vi "GraphZoom.vi"(7 "Plot":T1 items=["FRF", "rad phase unwrapped", "deg phase unwrapped", "rad phase wrapped", "deg phase wrapped", "White Plots", "MJ Map", "Real and Imaginary"], 9 "Names":string[](array[string]), 10 "dB Range":dbl=40.0, 11 "Graph":refnum<vi>) -> ()   [LabVIEW 2022 SP3]
uses:
  <vilib>/Utility/miscctls.llb/LVPoint32TypeDef.ctl
  GraphType.ctl
panel:
  out "option":bool
  in  "rescale Y":bool
  in  "View Type":u16(ring) items=["As measured"=0, "Normalize"=1, "Cplx Average"=3, "Real Average"=4]
  in  "Send Email":bool
  in  "Rescale":bool
  in  "Copy to Clipboard":bool
  out "Position":string
  in  "offset":bool
  in  "Plot grid":u32(colorbox)=16448250
  in  "Integrate":bool
  in  "Plot background":u32(colorbox)=16448250
  in  "Matlab":bool
  in  "Plot Format":T2
  in  "Separation":dbl=1.0
  in  "Separate":bool
  in  "Slide":dbl(slide) scale=-30.0..30.0
  in  "Run":u16(ring) items=["OB23BP_Starkie 04A H.AvC", "OB23_CurtinVLA Test 03 H.AvC"]
  out "lines":i32
  out "Data":cluster{dbl, "dt":dbl, "Y":dbl[]}[](graph)
  out "XScale.NameLbl.Text":string
  out "Coords":T3
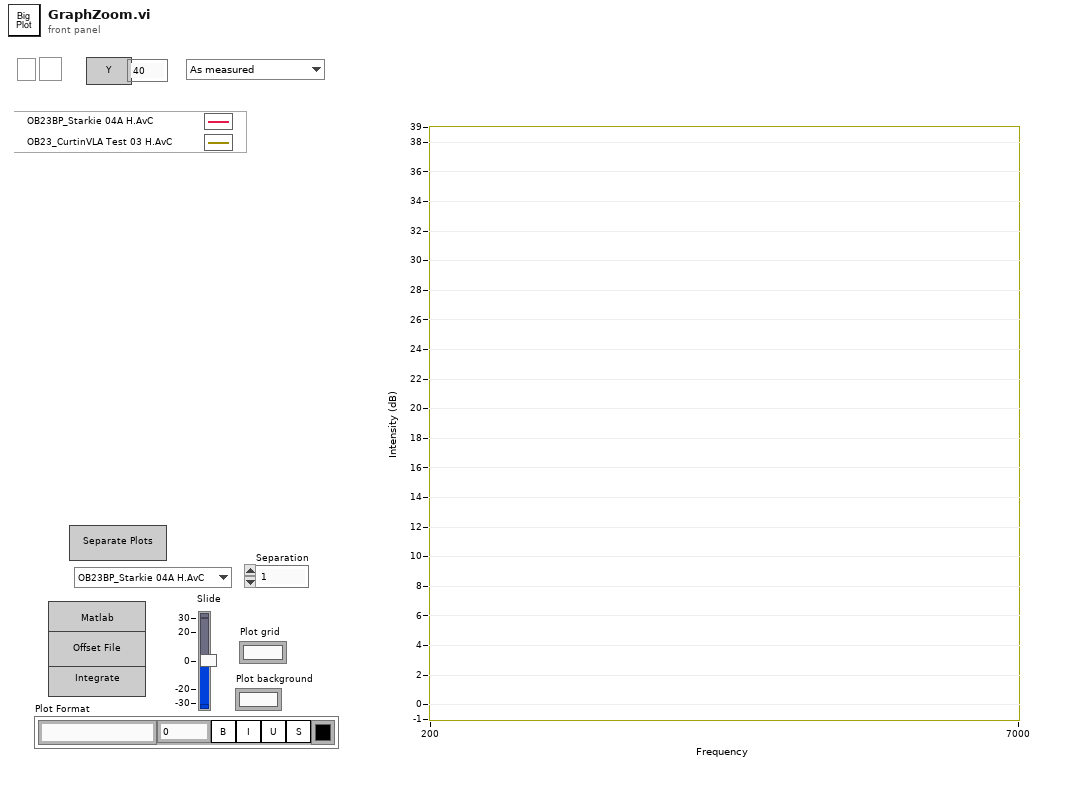
[diagram p1: front panel]
types:
  T1 = typedef "GraphType.ctl" = u16
  T2 = cluster{"Font Name":string, "Size":u16, "Bold":bool, "Italic":bool, "Underline":bool, "Strikeout":bool, "Color":u32}
  T3 = typedef "LVPoint32TypeDef.ctl" = cluster{"Horizontal":i32, "Vertical":i32}
  T4 = enum16{"Grab Lines", "Grab Bands", "Grab Centroids"}
  T5 = typedef "LVRangeTypeDef.ctl" = cluster{"Minimum":dbl, "Maximum":dbl, "Increment":dbl, "Minor Increment":dbl, "Start":dbl}
  T6 = typedef "LVFontTypeDef.ctl" = cluster{"Font Name":string, "Size":u16, "Bold":bool, "Italic":bool, "Underline":bool, "Strikeout":bool, "Color":u32}
  T7 = cluster{"View Type":u16, "Smoothing":u16, "Bands":u16, "New Band":bool, "rescale Y":bool, "rescale X":bool, "X_Low":dbl, "X_High":dbl, "dB Range":dbl, "New Band 2":bool, "X Scaling":bool, "Y Scaling":bool, "mag/phase":T1}
  T8 = cluster{"View Type":u16, "Smoothing":u16, "Bands":u16, "New Band":bool, "rescale Y":bool, "rescale X":bool, "X_Low":dbl, "X_High":dbl, "dB Range":dbl, "New Band 2":bool}
  T9 = cluster{"Shift":bool, "Ctrl":bool, "Alt":bool, "Cmd":bool, "Opt":bool}
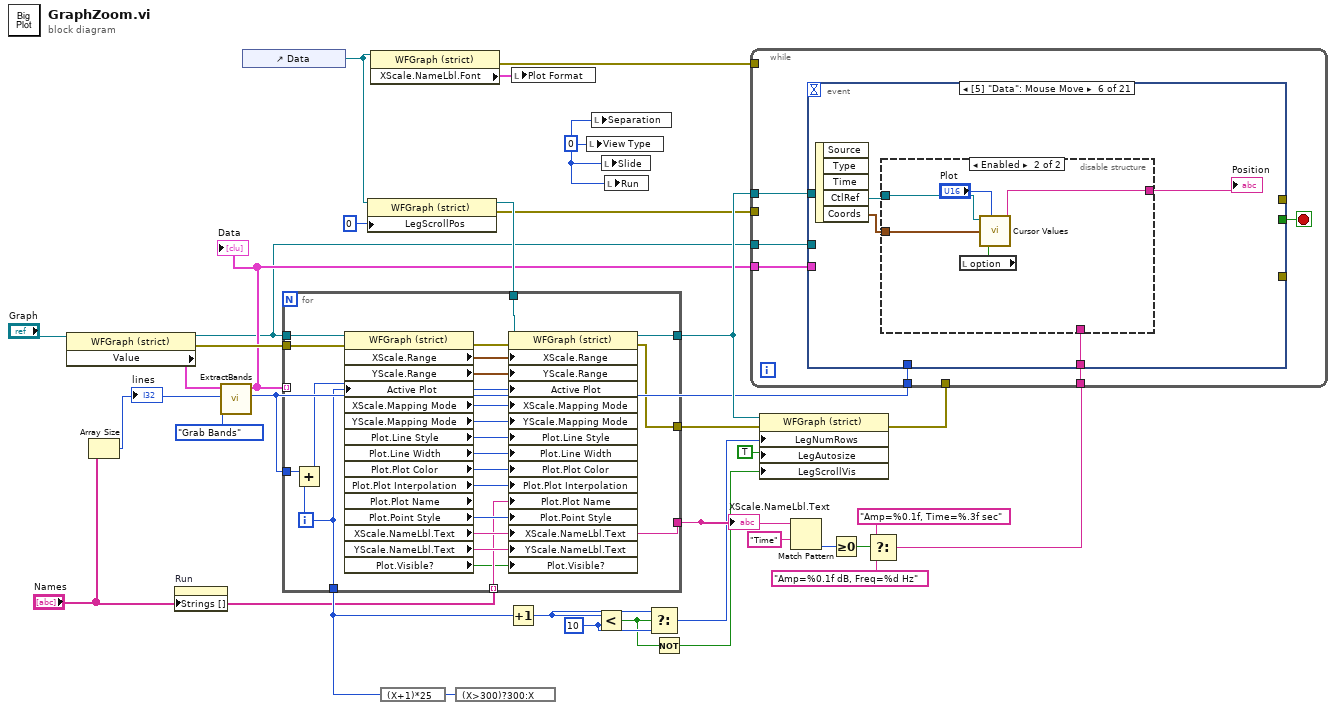
[diagram p0: block diagram]
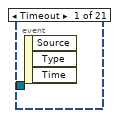
[diagram p2: hidden frame]
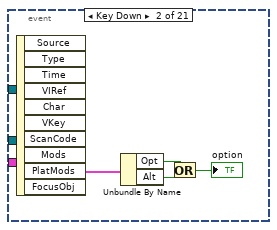
[diagram p3: hidden frame]
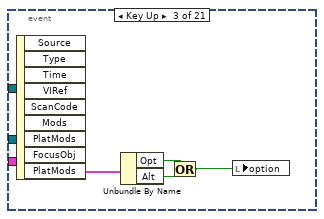
[diagram p4: hidden frame]
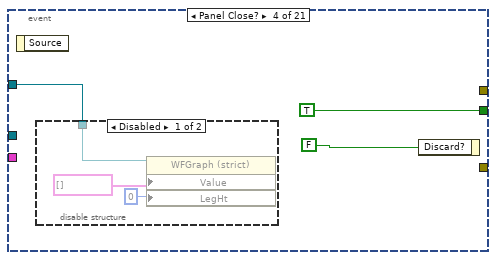
[diagram p5: hidden frame]
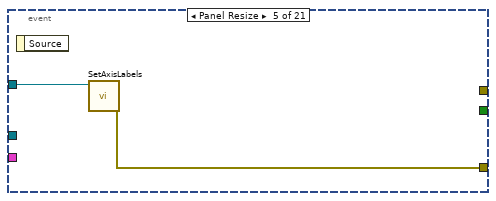
[diagram p7: hidden frame]
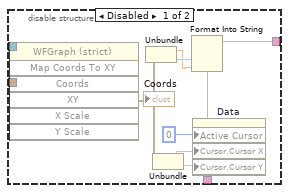
[diagram p8: hidden frame]
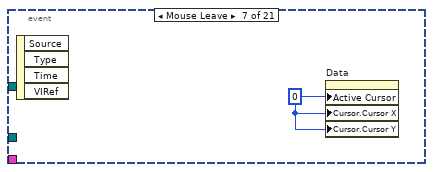
[diagram p9: hidden frame]
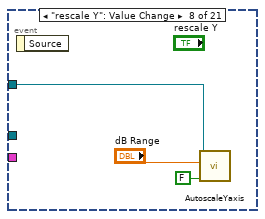
[diagram p10: hidden frame]
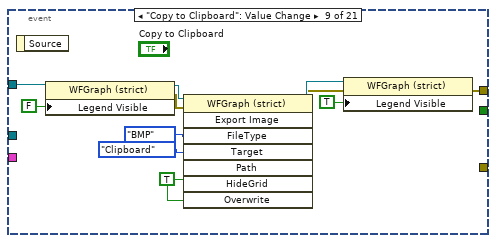
[diagram p11: hidden frame]
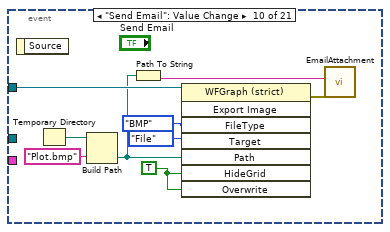
[diagram p12: hidden frame]
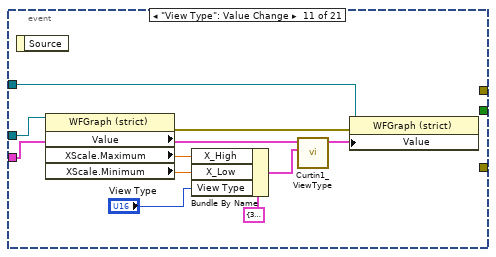
[diagram p13: hidden frame]
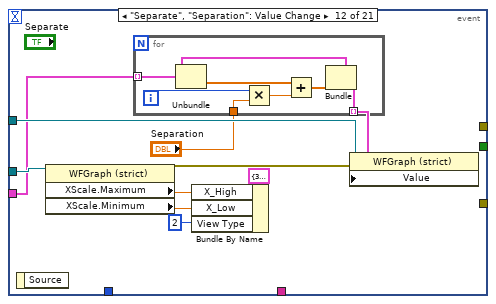
[diagram p14: hidden frame]
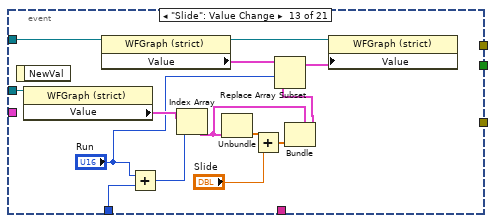
[diagram p15: hidden frame]
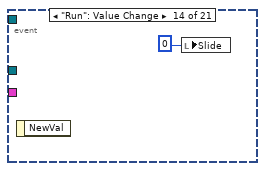
[diagram p16: hidden frame]
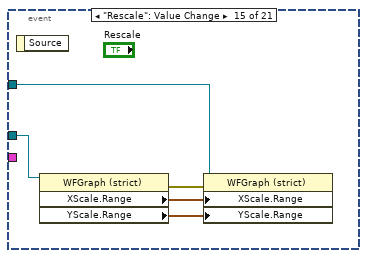
[diagram p17: hidden frame]
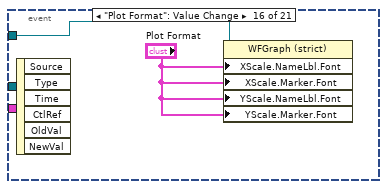
[diagram p18: hidden frame]
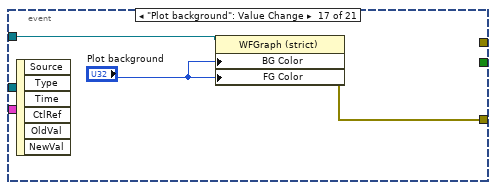
[diagram p19: hidden frame]
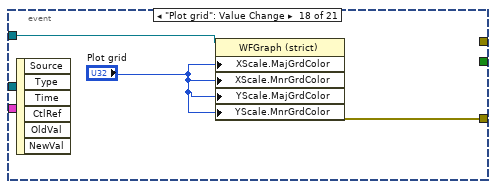
[diagram p20: hidden frame]
diagram:
  w16 = 10 ("y")
  w12 = 0
  n1 = property class="WFGraph (strict)"(reference="Graph") -> (reference out=w1:refnum<vi>, error out=w21:errorcluster, "Value"=w9:cluster{dbl, "dt":dbl, "Y":dbl[]}[])  [unwired: 1 in]
  n2 = Array Size(array="Names") -> (size(s)=w8:i32)
  "lines" <- w8
  n3 = property on="Run" class="Ring (strict)"("Strings []"="Names") -> ()  [unwired: 2 in, 2 out]
  n4 = call "ExtractBands.vi"("Task"=T4."Grab Bands", "lines"=w8, "plot in"=w9) -> ("Starting line"=w2:i32, "plot out"=w5:cluster{dbl, "dt":dbl, "Y":dbl[]}[])  [unwired: 7 in]
  "Data" <- w5
  n5 = control-ref of="Data"() -> (w6:refnum<vi>)
  n6 = property class="WFGraph (strict)"(reference=w6, "LegScrollPos"=u32 0 ("Legend:Scroll Position")) -> (reference out=w23:refnum<vi>, error out=w22:errorcluster)  [unwired: 1 in]
  n7 = for {
    tunnel: w1 -> [w53]
    tunnel: w23 -> [w52]
    tunnel: w5 -> [_] mode=indexing
    tunnel: [w35] -> w11
    tunnel: [w51] -> w26
    tunnel: [w43] -> w33
    tunnel: "Names" -> [w41] mode=indexing
    tunnel: w21 -> [w39]
    tunnel: [w38] -> w20
    tunnel: w2 -> [w37]
    i -> [w35]
    n8 = Add(x=w37, y=w35) -> (x+y=w36:i32)
    n9 = property class="WFGraph (strict)" props=["XScale", "Range", "YScale", "Range", "Active Plot", "XScale", "Mapping Mode", "YScale", "Mapping Mode", "Plot", "Line Style", "Plot", "Line Width", "Plot", "Plot Color", "Plot", "Plot Interpolation", "Plot", "Plot Name", "Plot", "Point Style", "XScale", "NameLbl", "Text", "YScale", "NameLbl", "Text", "Plot", "Visible?"](reference=w53, error in=w39, "Active Plot"=w36) -> (error out=w54:errorcluster, "XScale.Range"=w55:T5, "YScale.Range"=w56:T5, "XScale.Mapping Mode"=w50:u8, "YScale.Mapping Mode"=w49:u8, "Plot.Line Style"=w48:u8, "Plot.Line Width"=w47:u8, "Plot.Plot Color"=w46:u32, "Plot.Plot Interpolation"=w45:u8, "Plot.Point Style"=w44:u8, "XScale.NameLbl.Text"=w43:string, "YScale.NameLbl.Text"=w42:string, "Plot.Visible?"=w40:bool)  [unwired: 2 out]
    n10 = property class="WFGraph (strict)"(reference=w52, error in=w54, "XScale.Range"=w55, "YScale.Range"=w56, "Active Plot"=w35, "XScale.Mapping Mode"=w50, "YScale.Mapping Mode"=w49, "Plot.Line Style"=w48, "Plot.Line Width"=w47, "Plot.Plot Color"=w46, "Plot.Plot Interpolation"=w45, "Plot.Plot Name"=w41, "Plot.Point Style"=w44, "XScale.NameLbl.Text"=w43, "YScale.NameLbl.Text"=w42, "Plot.Visible?"=w40) -> (reference out=w51:refnum<vi>, error out=w38:errorcluster)
  }
  "XScale.NameLbl.Text" <- w33
  n11 = property class="WFGraph (strict)"(reference=w6) -> (error out=w3:errorcluster, "XScale.NameLbl.Font"=w18:T6)  [unwired: 1 in, 1 out]
  n12 = expression code="(X+1)*25"(w11) -> (w17:i32)
  n13 = expression code="(X>300)?300:X"(w17) -> ()  [unwired: 1 out]
  n14 = Increment(x=w11) -> (x+1=w10:i32)
  n15 = local write "Plot Format"(w18) -> ()
  n16 = local write "View Type"(w12) -> ()
  n17 = local write "Separation"(w12) -> ()
  n18 = Less?(x=w10, y=w16) -> (x < y?=w14:bool)
  n19 = local write "Slide"(w12) -> ()
  n20 = local write "Run"(w12) -> ()
  n21 = Select(t=w10, s=w14, f=w16) -> (s? t:f=w15:i32)
  n22 = Not(x=w14) -> (.not. x?=w13:bool)
  n23 = property class="WFGraph (strict)"(reference=w26, error in=w20, "LegNumRows"=w15, "LegAutosize"=TRUE ("Legend:Autosize"), "LegScrollVis"=w13) -> (error out=w19:errorcluster)  [unwired: 1 out]
  n24 = Match Pattern(string=w33, regular expression="Time") -> (offset past match=w31:i32)  [unwired: 1 in, 3 out]
  n25 = Greater Or Equal To 0?(x=w31) -> (x >= 0?=w30:bool)
  n26 = Select(t="Amp=%0.1f, Time=%.3f sec" ("format string"), s=w30, f="Amp=%0.1f dB, Freq=%d Hz" ("format string")) -> (s? t:f=w27:string)
  n27 = while {
    tunnel: w26 -> [w61]
    tunnel: w27 -> [w60]
    tunnel: w1 -> [w59]
    tunnel: w22 -> [_]
    tunnel: w19 -> [_]
    tunnel: w5 -> [w58]
    tunnel: w2 -> [w57]
    tunnel: w3 -> [_]
    stop <- w62 stop-if-true
    n28 = event shown="[5] \"Data\": Mouse Move" {
      selector: _ -> [_ _ _ _ _ _ _ _ _ _ _ _ _ _ _ _ _ _ _ _ _]
      dyn-events: _ -> [_ _ _ _ _ _ _ _ _ _ _ _ _ _ _ _ _ _ _ _ _]
      timeout: _ -> [_ _ _ _ _ _ _ _ _ _ _ _ _ _ _ _ _ _ _ _ _]
      tunnel: [_ _ _ TRUE ("Stop Button") _ _ _ _ _ _ _ _ _ _ _ _ _ _ _ _ _] -> w62
      tunnel: w61 -> [_ _ _ w73 w78 _ _ w101 w110 w119 w131 w141 w157 _ w165 w169 w173 w176 _ w180 _]
      tunnel: w60 -> [_ _ _ _ _ w80 _ _ _ _ _ _ _ _ _ _ _ _ _ _ _]
      tunnel: w59 -> [_ _ _ _ _ _ _ _ _ _ w128 w137 w162 _ w164 _ _ _ _ _ w191]
      tunnel: w58 -> [_ _ _ _ _ _ _ _ _ _ w124 w134 _ _ _ _ _ _ _ w178 _]
      tunnel: w57 -> [_ _ _ _ _ _ _ _ _ _ _ _ w149 _ _ _ _ _ _ _ w190]
      tunnel: [_ _ _ _ w77 _ _ _ _ _ _ _ _ _ _ _ w172 w175 _ _ _] -> _
      tunnel: [_ _ _ _ _ _ _ _ w102 _ _ _ _ _ _ _ _ _ _ _ _] -> _
      event Timeout {
        n29 = event-data() -> ()  [unwired: 1 in, 3 out]
      }
      event Key Down {
        n30 = event-data() -> ("PlatMods"=w66:T9)  [unwired: 1 in, 9 out]
        n31 = Unbundle By Name(w66) -> ("Opt"=w64:bool, "Alt"=w65:bool)
        n32 = Or(x=w64, y=w65) -> (x .or. y?=→"option":bool)
      }
      event Key Up {
        n33 = event-data() -> ("PlatMods"=w70:T9)  [unwired: 1 in, 8 out]
        n34 = Unbundle By Name(w70) -> ("Opt"=w68:bool, "Alt"=w69:bool)
        n35 = Or(x=w68, y=w69) -> (x .or. y?=w67:bool)
        n36 = local write "option"(w67) -> ()
      }
      event Panel Close? {
        n37 = event-data() -> ()  [unwired: 1 in, 1 out]
        n38 = disable-structure shown="Disabled" {
          disable-tunnel: w73 -> [w75 _]
          frame Disabled {
            n39 = property class="WFGraph (strict)"(reference=w75, "Value"=cluster{dbl, "dt":dbl, "Y":dbl[]}[] [], "LegHt"=u32 0 ("Legend:Size:Height")) -> ()  [unwired: 1 in, 2 out]
          }
          frame Enabled {
          }
        }
        n40 = event-data("Discard?"=FALSE) -> ()  [unwired: 1 in, 1 out]
      }
      event Panel Resize {
        n41 = event-data() -> ()  [unwired: 1 in, 1 out]
        n42 = call "SetAxisLabels.vi"("WaveformGraph in"=w78) -> ("error out"=w77:errorcluster)  [unwired: 8 in, 2 out]
      }
      event "Data": Mouse Move {
        n43 = event-data() -> ("CtlRef"=w79:refnum<vi>, "Coords"=w82:T3)  [unwired: 1 in, 3 out]
        n44 = disable-structure shown="Enabled" {
          disable-tunnel: w82 -> [w92 w94]
          disable-tunnel: [w91 w95] -> w81
          disable-tunnel: w80 -> [w84 _]
          disable-tunnel: w79 -> [w83 w96]
          frame Disabled {
            n45 = invoke class="WFGraph (strict)" method="Map Coords To XY"(reference=w83, "Coords"=w92) -> ("XY"=w87:cluster{"X":dbl, "Y":dbl})  [unwired: 5 in, 6 out]
            "Coords" <- w87
            n46 = Unbundle(w87) -> ("X"=w89:dbl, "Y"=w90:dbl)
            n47 = Unbundle(w87) -> ("X"=w86:dbl, "Y"=w85:dbl)
            n48 = Format Into String(format string=w84, w90, w89) -> (resulting string=w91:string)  [unwired: 2 in, 1 out]
            n49 = property on="Data" class="WFGraph (strict)"("Active Cursor"=u32 0, "Cursor.Cursor X"=w86, "Cursor.Cursor Y"=w85) -> ()  [unwired: 2 in, 2 out]
          }
          frame Enabled {
            n50 = local read "option"() -> (w97:bool)
            n51 = call "Cursor Values.vi"("Plot"="Plot", "option?"=w97, "Coords"=w94, "WaveformGraph in"=w96) -> ("Position"=w95:string)  [unwired: 7 in]
          }
        }
        "Position" <- w81
      }
      event Mouse Leave {
        w98 = u32 0 ("Active Cursor")
        n52 = event-data() -> ()  [unwired: 1 in, 4 out]
        n53 = property on="Data" class="WFGraph (strict)"("Active Cursor"=w98, "Cursor.Cursor X"=w98, "Cursor.Cursor Y"=w98) -> ()  [unwired: 2 in, 2 out]
      }
      event "rescale Y": Value Change {
        n54 = event-data() -> ()  [unwired: 1 in, 1 out]
        n55 = call "AutoscaleYaxis.vi"("Has Coherence in plot?"=FALSE, "dB Range"="dB Range", "WaveformGraph in"=w101) -> ()  [unwired: 9 in]
      }
      event "Copy to Clipboard": Value Change {
        w109 = TRUE ("Hide Grid")
        n56 = event-data() -> ()  [unwired: 1 in, 1 out]
        n57 = property class="WFGraph (strict)"(reference=w110, "Legend Visible"=FALSE ("Legend:Visible")) -> (reference out=w108:refnum<vi>, error out=w104:errorcluster)  [unwired: 1 in]
        n58 = invoke class="WFGraph (strict)" method="Export Image"(reference=w108, error in=w104, "FileType"=enum32{"BMP", "EPS", "EMF", "PICT"}."BMP" ("File Type"), "Target"=enum32{"File", "Clipboard"}."Clipboard", "HideGrid"=w109, "Overwrite"=w109) -> (reference out=w105:refnum<vi>, error out=w103:errorcluster)  [unwired: 2 in, 6 out]
        n59 = property class="WFGraph (strict)"(reference=w105, error in=w103, "Legend Visible"=TRUE ("Legend:Visible")) -> (error out=w102:errorcluster)  [unwired: 1 out]
      }
      event "Send Email": Value Change {
        w116 = TRUE ("Hide Grid")
        n60 = event-data() -> ()  [unwired: 1 in, 1 out]
        n61 = Temporary Directory() -> (w118:path)
        n62 = Build Path(base path=w118, name or relative path="Plot.bmp") -> (appended path=w114:path)
        n63 = Path To String(path=w114) -> (string=w115:string)
        n64 = invoke class="WFGraph (strict)" method="Export Image"(reference=w119, "FileType"=enum32{"BMP", "EPS", "EMF", "PICT"}."BMP" ("File Type"), "Target"=enum32{"File", "Clipboard"}."File", "Path"=w114, "HideGrid"=w116, "Overwrite"=w116) -> (error out=w113:errorcluster)  [unwired: 2 in, 7 out]
        n65 = call "EmailAttachment.vi"("error in (no error)"=w113, "Attachment path"=w115) -> ()  [unwired: 10 in]
      }
      event "View Type": Value Change {
        n66 = event-data() -> ()  [unwired: 1 in, 1 out]
        n67 = property class="WFGraph (strict)" props=["Value", "XScale", "Maximum", "XScale", "Minimum"](reference=w128) -> (error out=w130:errorcluster, "XScale.Maximum"=w127:dbl, "XScale.Minimum"=w126:dbl)  [unwired: 1 in, 2 out]
        n68 = Bundle By Name(cluster=T7 {"View Type"=3, "Smoothing"=0, "Bands"=0, "New Band"=FALSE, "rescale Y"=FALSE, "rescale X"=FALSE, "X_Low"=200.0, "X_High"=10000.0, "dB Range"=40.0, "New Band 2"=FALSE, "X Scaling"=FALSE, "Y Scaling"=FALSE, "mag/phase"=0} ("Settings"), "X_High"=w127, "X_Low"=w126, "View Type"="View Type") -> (w125:T7)
        n69 = call "Curtin1_ViewType.vi"("Settings"=w125, "FRF in"=w124) -> ("FRF Out"=w123:cluster{dbl, "df":dbl, dbl[]}[])  [unwired: 8 in, 1 out]
        n70 = property class="WFGraph (strict)"(reference=w131, error in=w130, "Value"=w123) -> ()  [unwired: 2 out]
      }
      event "Separate", "Separation": Value Change {
        n71 = event-data() -> ()  [unwired: 1 in, 1 out]
        n72 = property class="WFGraph (strict)"(reference=w137) -> (error out=w140:errorcluster, "XScale.Maximum"=w136:dbl, "XScale.Minimum"=w135:dbl)  [unwired: 1 in, 1 out]
        n73 = for {
          tunnel: w134 -> [w147] mode=indexing
          tunnel: "Separation" -> [w143]
          tunnel: [w145] -> w132 mode=indexing
          i -> [w144]
          n74 = Unbundle(w147) -> ("Y"=w148:dbl[])  [unwired: 2 out]
          n75 = Multiply(x=w144, y=w143) -> (x*y=w142:dbl)
          n76 = Add(x=w148, y=w142) -> (x+y=w146:dbl[])
          n77 = Bundle(cluster=w147, "Y"=w146) -> (w145:cluster{dbl, "dt":dbl, "Y":dbl[]})  [unwired: 2 in]
        }
        n78 = Bundle By Name(cluster=T8 {"View Type"=3, "Smoothing"=0, "Bands"=0, "New Band"=FALSE, "rescale Y"=FALSE, "rescale X"=FALSE, "X_Low"=200.0, "X_High"=10000.0, "dB Range"=40.0, "New Band 2"=FALSE} ("Settings"), "X_High"=w136, "X_Low"=w135, "View Type"=u16 2) -> ()  [unwired: 1 out]
        n79 = property class="WFGraph (strict)"(reference=w141, error in=w140, "Value"=w132) -> ()  [unwired: 2 out]
      }
      event "Slide": Value Change {
        n80 = event-data() -> ()  [unwired: 1 in, 1 out]
        n81 = property class="WFGraph (strict)"(reference=w162) -> ("Value"=w159:cluster{dbl, "dt":dbl, "Y":dbl[]}[])  [unwired: 1 in, 2 out]
        n82 = property class="WFGraph (strict)"(reference=w157) -> (reference out=w153:refnum<vi>, "Value"=w156:cluster{dbl, "dt":dbl, "Y":dbl[]}[])  [unwired: 1 in, 1 out]
        n83 = Add(x="Run", y=w149) -> (x+y=w150:i32)
        n84 = Index Array(array=w159, index=w150) -> (element=w158:cluster{dbl, "dt":dbl, "Y":dbl[]})
        n85 = Unbundle(w158) -> ("Y"=w161:dbl[])  [unwired: 2 out]
        n86 = Add(x=w161, y="Slide") -> (x+y=w160:dbl[])
        n87 = Bundle(cluster=w158, "Y"=w160) -> (w155:cluster{dbl, "dt":dbl, "Y":dbl[]})  [unwired: 2 in]
        n88 = Replace Array Subset(array=w156, new element=w155, index="Run") -> (w154:cluster{dbl, "dt":dbl, "Y":dbl[]}[])
        n89 = property class="WFGraph (strict)"(reference=w153, "Value"=w154) -> ()  [unwired: 1 in, 2 out]
      }
      event "Run": Value Change {
        n90 = event-data() -> ()  [unwired: 1 in, 1 out]
        n91 = local write "Slide"(0) -> ()
      }
      event "Rescale": Value Change {
        n92 = event-data() -> ()  [unwired: 1 in, 1 out]
        n93 = property class="WFGraph (strict)"(reference=w164) -> (error out=w168:errorcluster, "XScale.Range"=w167:T5, "YScale.Range"=w166:T5)  [unwired: 1 in, 1 out]
        n94 = property class="WFGraph (strict)"(reference=w165, error in=w168, "XScale.Range"=w167, "YScale.Range"=w166) -> ()  [unwired: 2 out]
      }
      event "Plot Format": Value Change {
        n95 = event-data() -> ()  [unwired: 1 in, 6 out]
        n96 = property class="WFGraph (strict)"(reference=w169, "XScale.NameLbl.Font"="Plot Format", "XScale.Marker.Font"="Plot Format", "YScale.NameLbl.Font"="Plot Format", "YScale.Marker.Font"="Plot Format") -> ()  [unwired: 1 in, 2 out]
      }
      event "Plot background": Value Change {
        n97 = event-data() -> ()  [unwired: 1 in, 6 out]
        n98 = property class="WFGraph (strict)"(reference=w173, "BG Color"="Plot background", "FG Color"="Plot background") -> (error out=w172:errorcluster)  [unwired: 1 in, 1 out]
      }
      event "Plot grid": Value Change {
        n99 = event-data() -> ()  [unwired: 1 in, 6 out]
        n100 = property class="WFGraph (strict)"(reference=w176, "XScale.MajGrdColor"="Plot grid", "XScale.MnrGrdColor"="Plot grid", "YScale.MajGrdColor"="Plot grid", "YScale.MnrGrdColor"="Plot grid") -> (error out=w175:errorcluster)  [unwired: 1 in, 1 out]
      }
      event "Matlab": Value Change {
        n101 = event-data() -> ()  [unwired: 1 in, 1 out]
        n102 = control-ref of="Data"() -> (w177:refnum<vi>)
        n103 = call "MATLAB.vi"("Graph"=w177) -> ()  [unwired: 10 in, 1 out]
      }
      event "Integrate": Value Change {
        n104 = event-data() -> ()  [unwired: 1 in, 1 out]
        n105 = for {
          tunnel: [w183] -> w179 mode=indexing
          tunnel: w178 -> [w182] mode=indexing
          w181 = u16 1 items=["Accelerometer", "Accel (speed)", "Microphone", "Vibrometer"] ("Output")
          n106 = call "IntegrateFRF.vi"("Output"=w181, "Complex FRF"=w182) -> ("FRF out"=w183:cluster{"t0":dbl, "dt":dbl, dbl[]})  [unwired: 8 in, 1 out]
        }
        n107 = property class="WFGraph (strict)"(reference=w180, "Value"=w179) -> ()  [unwired: 1 in, 2 out]
      }
      event "offset": Value Change {
        n108 = event-data() -> ()  [unwired: 1 in, 1 out]
        n109 = local read "Run"() -> (w192:u16)
        n110 = property class="WFGraph (strict)"(reference=w191) -> ("Value"=w193:cluster{dbl, "dt":dbl, "Y":dbl[]}[])  [unwired: 1 in, 2 out]
        n111 = Add(x=w192, y=w190) -> (x+y=w194:i32)
        n112 = call "Curtin1_GlobalFolder.vi"() -> ("LabVIEW Data Path"=w185:path)  [unwired: 1 in, 1 out]
        n113 = Strip Path(path=w185) -> (stripped path=w184:path)  [unwired: 1 out]
        n114 = Index Array(array=w193, index=w194) -> (element=w189:cluster{dbl, "dt":dbl, "Y":dbl[]})
        n115 = call "File Dialog"("start path"=w184) -> ("selected path"=w188:path, "cancelled"=w187:bool, "error out"=w186:errorcluster)  [unwired: 11 in, 1 out]
        n116 = case shown="False" w187 {
          tunnel: w189 -> [w198 _]
          tunnel: w188 -> [w195 _]
          tunnel: w186 -> [_ _]
          frame False {
            n117 = call "SaveTSVFile.vi"("Task"=enum16{"Save Magnitude", "Save Complex"}."Save Magnitude", "type"=enum16{"tsv", "csv"}."tsv", "FRF"=w198, "Path"=w195) -> ()  [unwired: 7 in, 1 out]
          }
          frame True {
          }
        }
        n118 = disable-structure shown="Disabled" {
          frame Disabled {
            n119 = call "SaveStoppanniFile.vi"() -> ()  [unwired: 11 in, 1 out]
            n120 = call "Curtin1_Recalc.vi"() -> ()  [unwired: 12 in]
          }
          frame Enabled {
          }
        }
      }
    }
  }
